vi "Node.vi"(8 "error in (no error)":errorcluster, 11 "GroupAbstract in":refnum<class "GroupAbstract.lvclass">) -> (0 "error out":errorcluster, 2 "Node":string, 3 "GroupAbstract out":refnum<class "GroupAbstract.lvclass">)   [LabVIEW 2020, in "Vecto.lvlib" / "GroupAbstract.lvclass"]
uses:
  GroupAbstract.lvclass
  GroupAbstract.lvclass/GroupAbstract.ctl
  Group Config/Group Config.lvclass
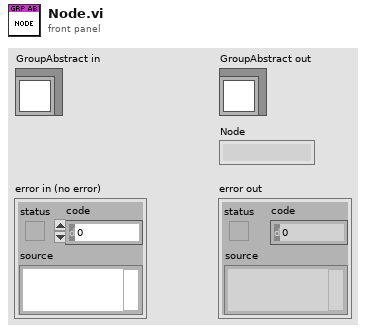
[diagram p1: front panel]
types:
  T1 = typedef "Vecto.lvlib/Group Info.ctl" = cluster{"System":string, "Cluster":string, "Node":string, "Task":string, "Name":string}
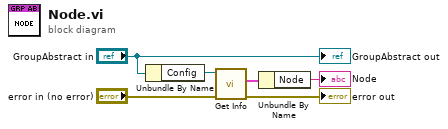
[diagram p0: block diagram]
diagram:
  n1 = Unbundle By Name("GroupAbstract in") -> ("Config"=w5:refnum<class "Group Config.lvclass">)
  n2 = call "Get Info.vi"("error in (no error)"="error in (no error)", "Group Config in"=w5) -> ("error out"=→"error out":errorcluster, "Info"=w4:T1)  [unwired: 7 in, 1 out]
  n3 = Unbundle By Name(w4) -> ("Node"=→"Node":string)
  "GroupAbstract out" <- "GroupAbstract in"
